vi "SNDCSDLM_LV2009_sample.vi"() -> ()   [LabVIEW 2015]
panel:
  out "error out":errorcluster
  out "error message":string
  in  "Error Code":i32 caption="error code (0)" format="%.0g"
  out "Current Measurement":dbl
  out "Voltage Measurement":dbl
  in  "Output State":bool=TRUE caption="State (Off)"
  in  "Voltage":dbl=14.4 caption="Voltage (0.0)"
  in  "Current":dbl=50.0 caption="Current (0.0)"
  in  "Error In":errorcluster {"code" format="%.0x"}
  in  "Reset Device":bool=TRUE caption="reset device (Yes)"
  in  "ID Query":bool=TRUE caption="id query (Yes)"
  in  "Resource Name":refnum<visa-resource-name>="GPIB0::7::INSTR" caption="resource name"
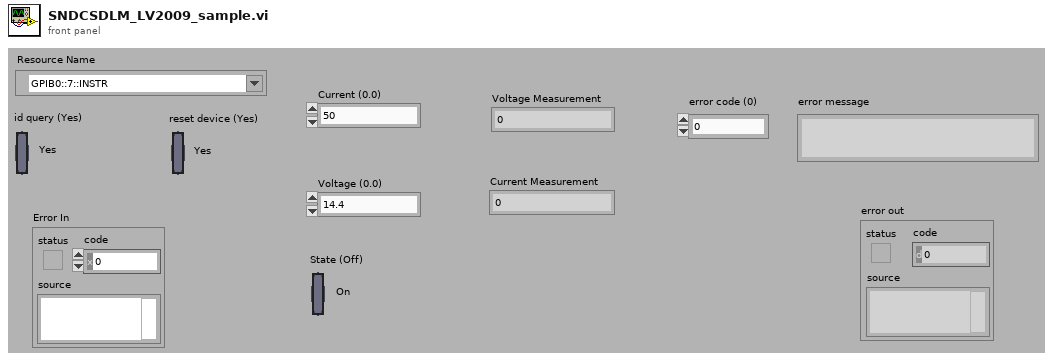
[diagram p1: front panel]
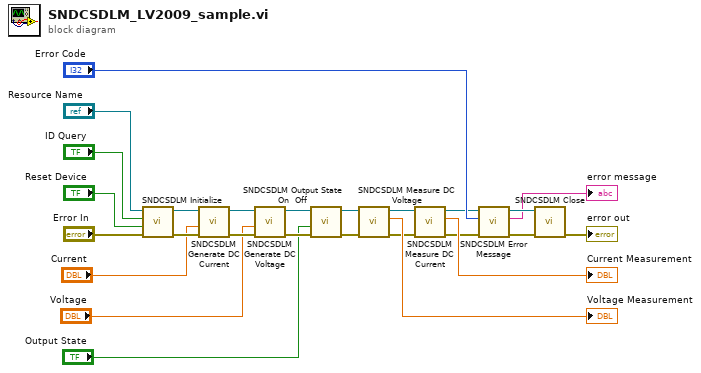
[diagram p0: block diagram]
diagram:
  n1 = call <instrlib>:"SNDCSDLM Initialize.vi"("error in (no error)"="Error In", "reset device (Yes)"="Reset Device", "id query (Yes)"="ID Query", "resource name"="Resource Name") -> ("error out"=w21:errorcluster, "instrument handle out"=w22:refnum<visa-resource-name>)  [unwired: 6 in]
  n2 = call <instrlib>:"SNDCSDLM Generate DC Current.vi"("error in (no error)"=w21, "Current (0.0)"="Current", "instrument handle"=w22) -> ("error out"=w15:errorcluster, "instrument handle out"=w16:refnum<visa-resource-name>)  [unwired: 7 in]
  n3 = call <instrlib>:"SNDCSDLM Generate DC Voltage.vi"("error in (no error)"=w15, "Voltage (0.0)"="Voltage", "instrument handle"=w16) -> ("error out"=w12:errorcluster, "instrument handle out"=w13:refnum<visa-resource-name>)  [unwired: 7 in]
  n4 = call <instrlib>:"SNDCSDLM Output State On  Off.vi"("error in (no error)"=w12, "State (Off)"="Output State", "instrument handle"=w13) -> ("error out"=w9:errorcluster, "instrument handle out"=w8:refnum<visa-resource-name>)  [unwired: 7 in]
  n5 = call <instrlib>:"SNDCSDLM Measure DC Voltage.vi"("error in (no error)"=w9, "instrument handle"=w8) -> ("error out"=w6:errorcluster, "Voltage Measurement"=→"Voltage Measurement":dbl, "instrument handle out"=w7:refnum<visa-resource-name>)  [unwired: 7 in]
  n6 = call "SNDCSDLM Measure DC Current.vi"("error in (no error)"=w6, "instrument handle"=w7) -> ("error out"=w2:errorcluster, "Current Measurement"=→"Current Measurement":dbl, "instrument handle out"=w1:refnum<visa-resource-name>)  [unwired: 7 in]
  n7 = call <instrlib>:"SNDCSDLM Error Message.vi"("error in (no error)"=w2, "error code (0)"="Error Code", "instrument handle"=w1) -> ("error out"=w19:errorcluster, "error message"=→"error message":string, "instrument handle out"=w20:refnum<visa-resource-name>)  [unwired: 6 in]
  n8 = call <instrlib>:"SNDCSDLM Close.vi"("error in (no error)"=w19, "instrument handle"=w20) -> ("error out"=→"error out":errorcluster)  [unwired: 9 in]
